vi "BrokenWhiteNoise.vi"() -> ()   [LabVIEW 2014]
uses:
  <vilib>/DAQmx/create/channels.llb/DAQmx Create Channel (AO-Voltage-Basic).vi
  <vilib>/DAQmx/write.llb/DAQmx Write (Analog Wfm 1Chan NSamp).vi
  <vilib>/measure/NI_MABase.lvlib
panel:
  out "Numeric":i32
  in  "Stop":bool
  out "White noise":errorcluster
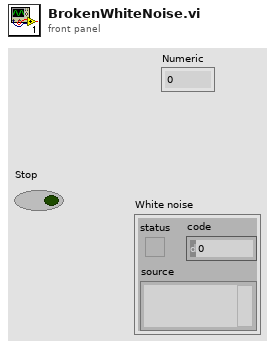
[diagram p1: front panel]
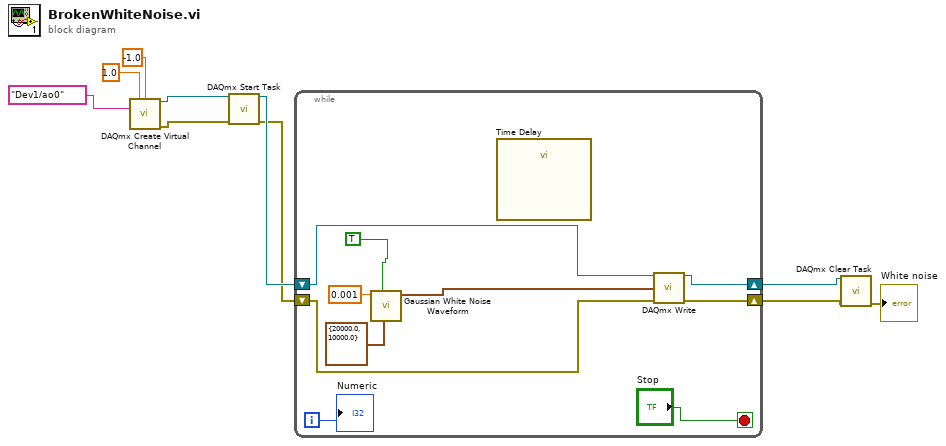
[diagram p0: block diagram]
diagram:
  n1 = call-poly <vilib>:"DAQmx Create Virtual Channel.vi"("maximum value"=1.0, "minimum value"=-1.0, "physical channels"=tag "Dev1/ao0") -> ("task out"=w7:refnum<k21>, "error out"=w5:errorcluster)  [unwired: 11 in]
  n2 = call <vilib>:"DAQmx Start Task.vi"("task/channels in"=w7, "error in"=w5) -> ("task out"=w6:refnum<k21>, "error out"=w4:errorcluster)  [unwired: 12 in]
  n3 = while {
    shift-right: [w16] -> w2
    shift-left: w6 -> [w18]
    shift-right: [w15] -> w1
    shift-left: w4 -> [w17]
    i -> [w12]
    stop <- "Stop" stop-if-true
    n4 = call <vilib>:"Gaussian White Noise Waveform.vi"("sampling info"=cluster{"Fs":dbl, "#s":dbl} {"Fs"=20000.0, "#s"=10000.0}, "reset signal"=TRUE, "standard deviation"=0.001) -> ("signal out"=w11:waveform(dbl))  [unwired: 7 in, 1 out]
    n5 = call "Time Delay"() -> ()  [unwired: 11 in, 1 out]
    n6 = call-poly <vilib>:"DAQmx Write.vi"("task/channels in"=w18, "data"=w11, "error in"=w17) -> ("task out"=w16:refnum<k21>, "error out"=w15:errorcluster)  [unwired: 10 in, 1 out]
    "Numeric" <- w12
  }
  n7 = call <vilib>:"DAQmx Clear Task.vi"("task in"=w2, "error in"=w1) -> ("error out"=→"White noise":errorcluster)  [unwired: 13 in]
